vi "PDM Acq Cfg Popup.vi"(8 "error in (no error)":errorcluster, 11 "config file in":path caption="Configuration File") -> (0 "error out":errorcluster, 2 "output setting":T3={"PDM clock rate"=3072000.0, "decimation factor"=64, "bit clock direction"=enum."In", "logic level"=enum."3.3 V"} {"decimation factor" items=["24"=24, "32"=32, "48"=48, "64"=64, "96"=96, "128"=128]; "PDM clock rate" format="%#_6p"}, 3 "config file out":path caption="Configuration File")   [LabVIEW 2022 SP3, in "Config Dialog.lvlib"]
uses:
  Config Dialog.lvlib
  controls/PDM/PDM input settings.ctl
  <vilib>/PDM Acquisition Toolkit/shared/controls/decimation order.ctl
  controls/bit clock direction.ctl
  <vilib>/PDM Acquisition Toolkit/host/Classes/Session/Controls/Logic Levels.ctl
  controls/logic level.ctl
  <vilib>/Utility/miscctls.llb/LVPointTypeDef.ctl
  <vilib>/PDM Acquisition Toolkit/shared/PDM Shared.lvlib
  <vilib>/PDM Acquisition Toolkit/host/Classes/Session/DecoderSession.lvclass
  input configuration file/input cfg file.lvlib
  input configuration file/PDM/PDM input cfg file.lvlib
panel:
  out "bit clock rate":dbl=25600.0 caption="Bit Clock Rate" format="%#_6pS/s"
  in  "Logic Level":T1
  in  "Decimation":u16(ring) caption="master clock source" items=["x24"=24, "x32"=32, "x48"=48, "x64"=64, "x96"=96, "x128"=128]
  in  "Bit Clock Direction":T2 caption="master clock source"
  in  "sample rate":dbl=25600.0 caption="Sampling rate" format="%#_6pS/s"
  in  "Save":bool
  # "PDM Input Configuration"
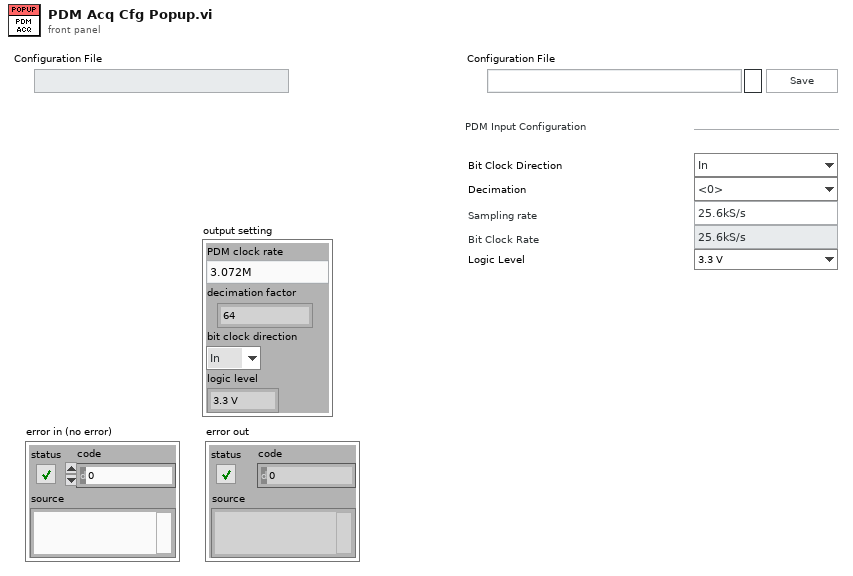
[diagram p1: front panel]
types:
  T1 = typedef "logic level.ctl" = enum32{"3.3 V", "1.8 V", "1.2 V"}
  T2 = typedef "bit clock direction.ctl" = enum32{"In", "Out"}
  T3 = typedef "PDM input settings.ctl" = cluster{"PDM clock rate":dbl, "decimation factor":T4, "bit clock direction":T2, "logic level":T5}
  T4 = typedef "PDM Shared.lvlib/decimation order.ctl" = u16
  T5 = typedef "PDM Acquisition Class Library.lvlib/DecoderSession.lvclass/Logic Levels.ctl" = enum16{"3.3 V", "1.8 V", "1.2 V"}
  T6 = typedef "LVPointTypeDef.ctl" = cluster{"Horizontal":i16, "Vertical":i16}
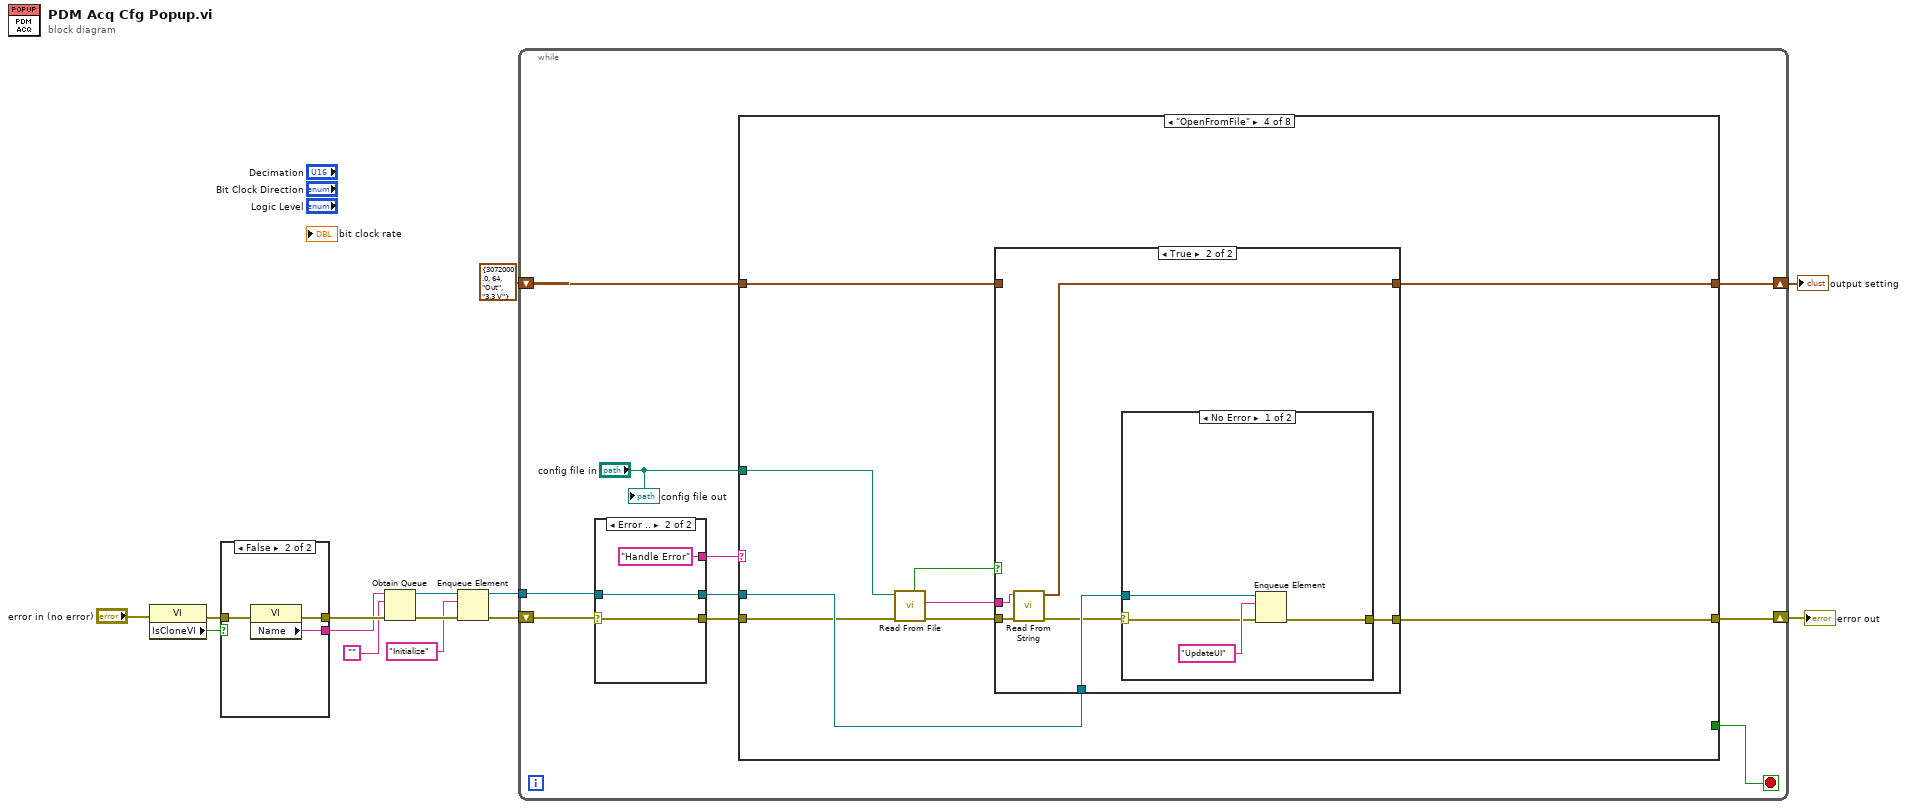
[diagram p0: block diagram]
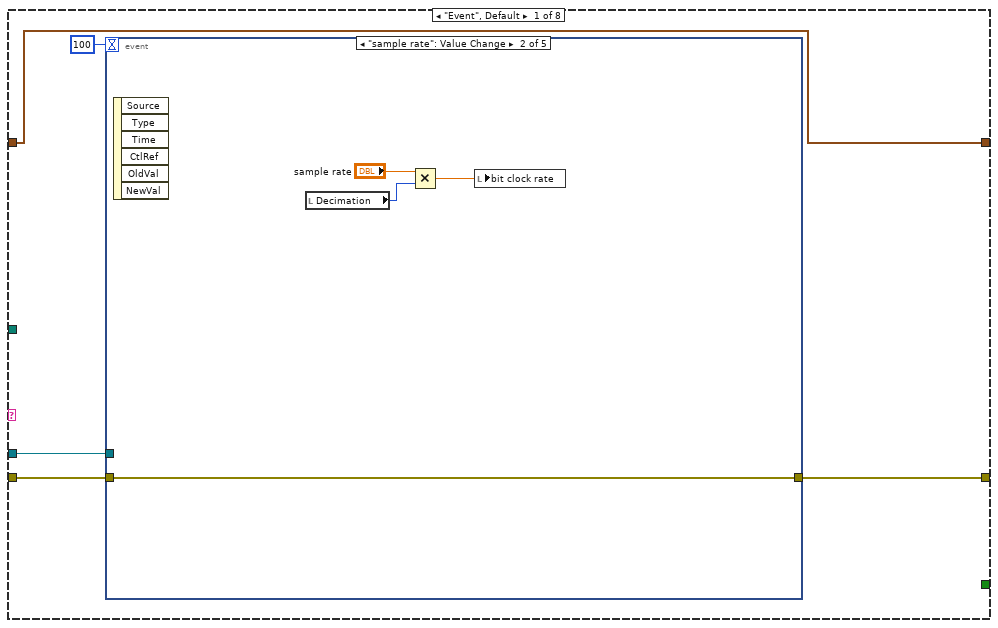
[diagram p2: hidden frame]
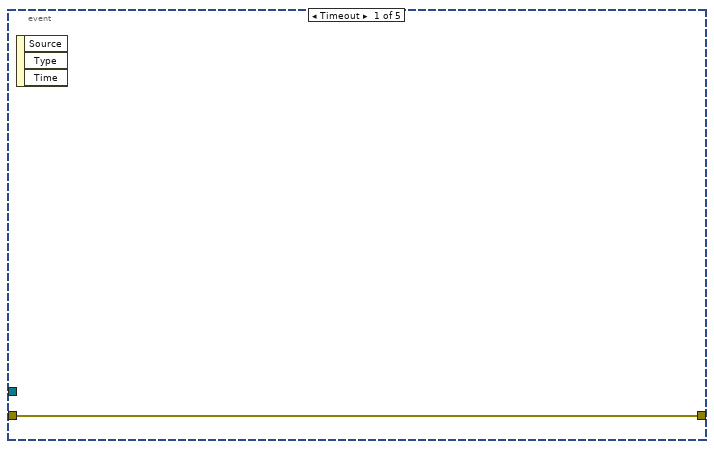
[diagram p3: hidden frame]
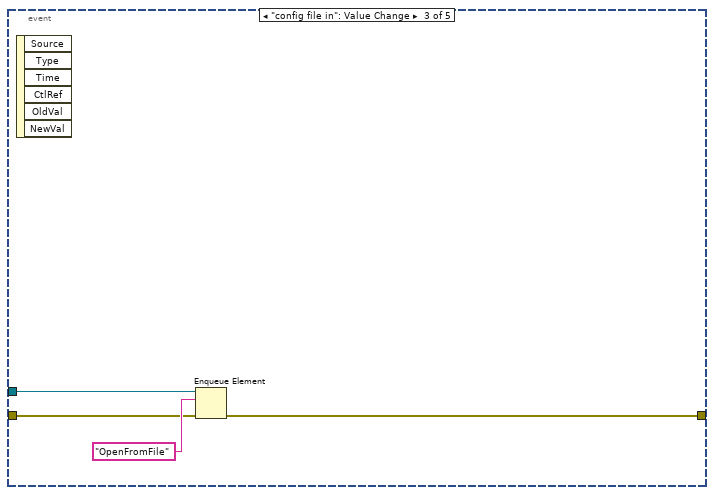
[diagram p4: hidden frame]
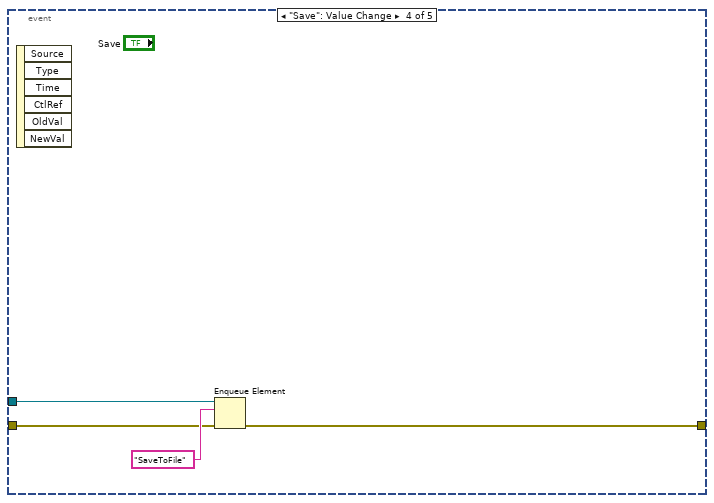
[diagram p5: hidden frame]
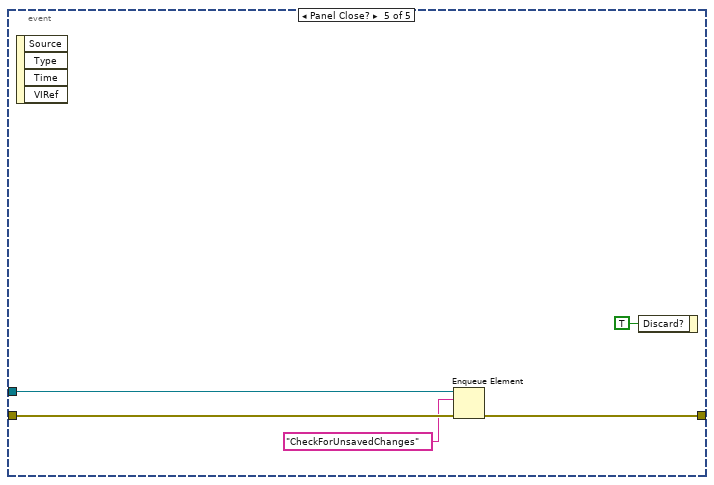
[diagram p6: hidden frame]
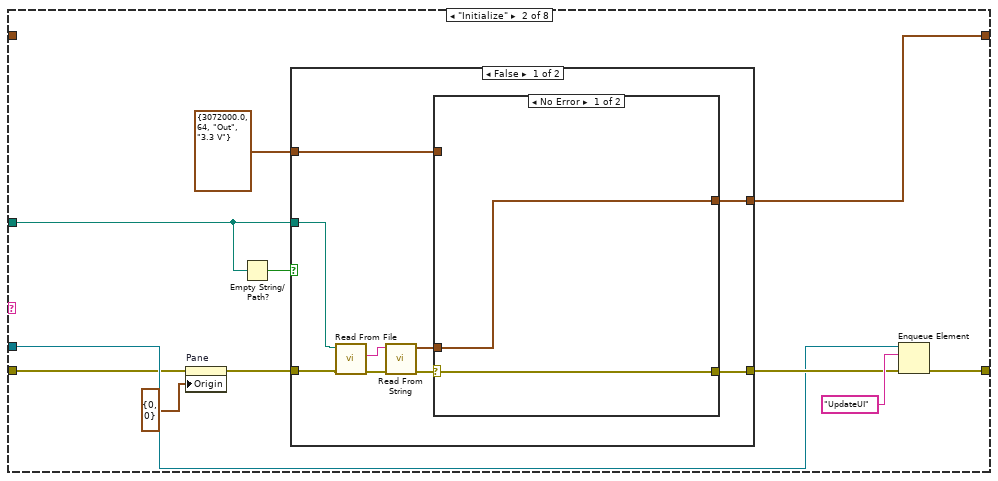
[diagram p7: hidden frame]
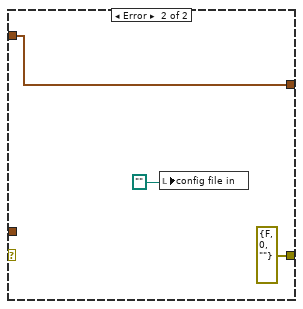
[diagram p8: hidden frame]
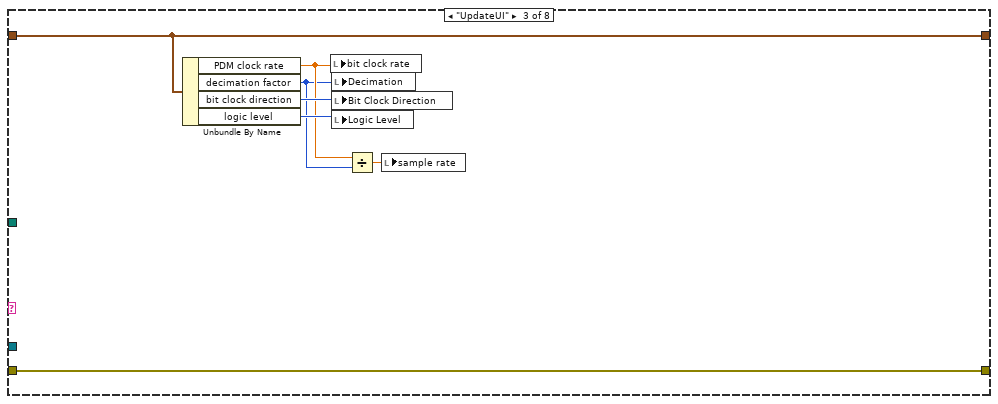
[diagram p10: hidden frame]
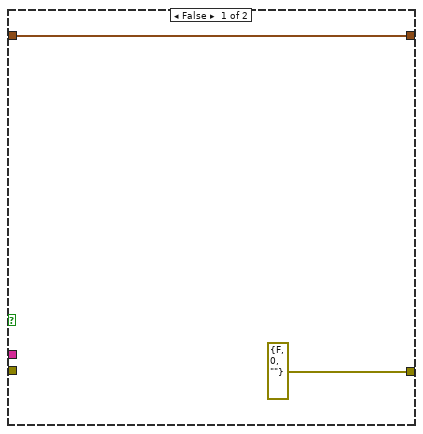
[diagram p11: hidden frame]
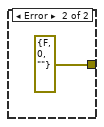
[diagram p12: hidden frame]
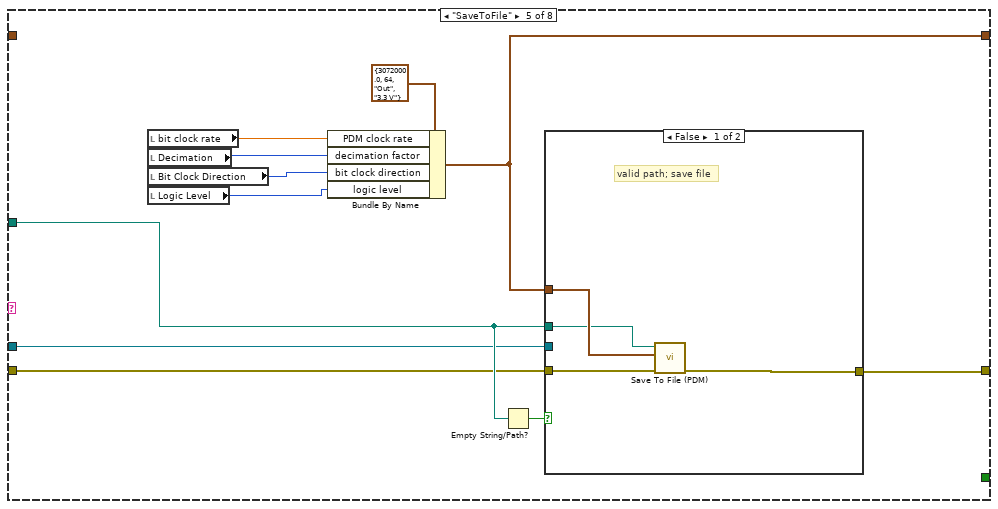
[diagram p13: hidden frame]
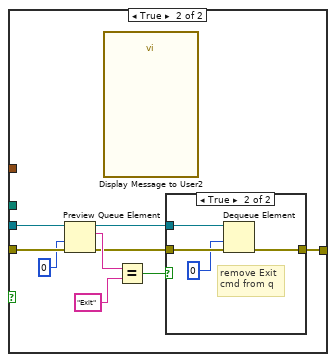
[diagram p14: hidden frame]
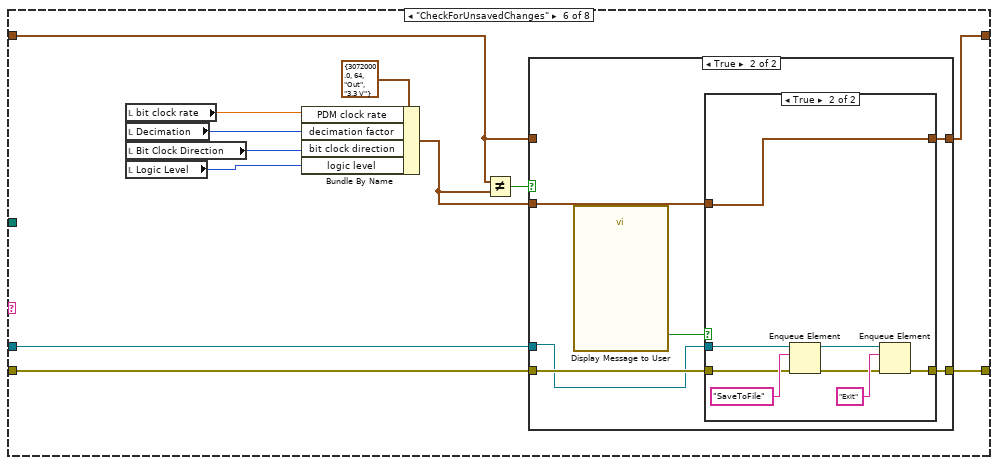
[diagram p16: hidden frame]
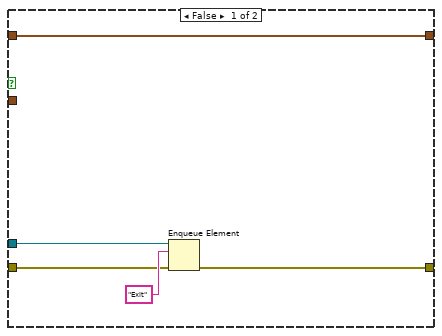
[diagram p17: hidden frame]
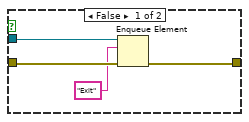
[diagram p18: hidden frame]
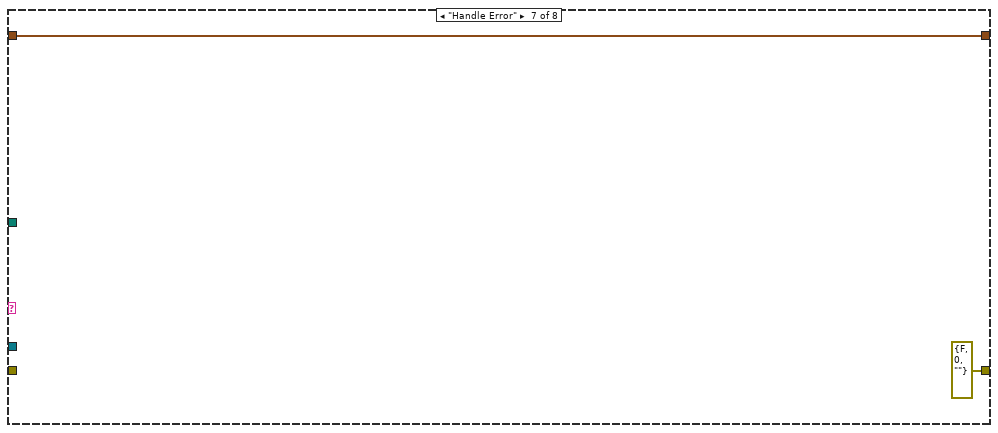
[diagram p19: hidden frame]
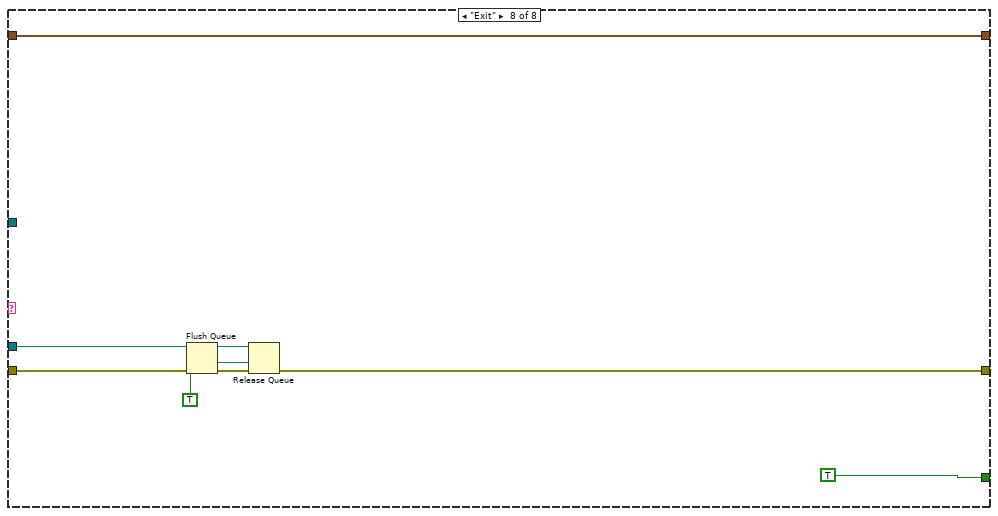
[diagram p20: hidden frame]
diagram:
  n1 = property class="VI"(error in="error in (no error)") -> (error out=w7:errorcluster, "IsCloneVI"=w8:bool)  [unwired: 1 in, 1 out]
  n2 = case shown="False" w8 {
    tunnel: [w17 w20] -> w14
    tunnel: [w16 w19] -> w13
    tunnel: w7 -> [w15 w18]
    frame True {
      n3 = property class="VI"(error in=w15) -> (error out=w17:errorcluster, "Clone Name"=w16:string)  [unwired: 1 in, 1 out]
    }
    frame False {
      n4 = property class="VI"(error in=w18) -> (error out=w20:errorcluster, "Name"=w19:string)  [unwired: 1 in, 1 out]
    }
  }
  n5 = Obtain Queue(name (unnamed)=w13, element data type="", error in (no error)=w14) -> (queue out=w11:refnum<queue>, error out=w12:errorcluster)  [unwired: 2 in, 1 out]
  n6 = Enqueue Element(queue=w11, element="Initialize", error in (no error)=w12) -> (queue out=w5:refnum<queue>, error out=w6:errorcluster)  [unwired: 1 in, 1 out]
  n7 = while {
    tunnel: w5 -> [w29]
    shift-right: [w25] -> w4
    shift-left: w6 -> [w30]
    shift-right: [w22] -> w1
    shift-left: T3 {"PDM clock rate"=3072000.0, "decimation factor"=64, "bit clock direction"=enum."Out", "logic level"=enum."3.3 V"} ("PDM input settings") -> [w23]
    stop <- w24 stop-if-true
    n8 = case shown="Error .." w30 {
      selector: w30 -> [w189 w192]
      tunnel: [w188 w192] -> w26
      tunnel: w29 -> [w187 w191]
      tunnel: [w186 w191] -> w27
      tunnel: [w185 "Handle Error"] -> w28
      frame No Error {
        n9 = Dequeue Element(queue=w187, timeout in ms (-1)=100, error in (no error)=w189) -> (queue out=w186:refnum<queue>, element=w185:string, error out=w188:errorcluster)  [unwired: 1 out]
      }
      frame Error {
      }
    }
    n10 = case shown="\"OpenFromFile\"" w28 {
      tunnel: w27 -> [w33 w58 _ w96 w115 w146 _ w179]
      tunnel: w26 -> [w34 w56 w87 w92 w117 w149 _ w180]
      tunnel: [w32 w59 w87 w95 w120 w148 errorcluster {"status"=FALSE, "code"=0, "source"=""} ("error out") w177] -> w25
      tunnel: [_ _ _ _ _ _ _ TRUE] -> w24
      tunnel: w23 -> [w31 _ w86 w94 _ w144 w175 w176]
      tunnel: [w31 w62 w86 w93 w119 w147 w175 w176] -> w22
      tunnel: "config file in" -> [_ w63 _ w91 w118 _ _ _]
      frame "Event", Default {
        n11 = event shown="[1] \"sample rate\": Value Change" {
          selector: _ -> [_ _ _ _ _]
          dyn-events: _ -> [_ _ _ _ _]
          timeout: 100 -> [_ _ _ _ _]
          tunnel: w34 -> [w36 w37 w43 w47 w52]
          tunnel: w33 -> [_ _ w42 w46 w51]
          tunnel: [w36 w37 w41 w45 w50] -> w32
          event Timeout {
            n12 = event-data() -> ()  [unwired: 1 in, 3 out]
          }
          event "sample rate": Value Change {
            n13 = event-data() -> ()  [unwired: 1 in, 6 out]
            n14 = local read "Decimation"() -> (w39:u16)
            n15 = Multiply(x="sample rate", y=w39) -> (x*y=w38:dbl)
            n16 = local write "bit clock rate"(w38) -> ()
          }
          event "config file in": Value Change {
            n17 = event-data() -> ()  [unwired: 1 in, 6 out]
            n18 = Enqueue Element(queue=w42, element="OpenFromFile", error in (no error)=w43) -> (error out=w41:errorcluster)  [unwired: 1 in, 2 out]
          }
          event "Save": Value Change {
            n19 = event-data() -> ()  [unwired: 1 in, 6 out]
            n20 = Enqueue Element(queue=w46, element="SaveToFile", error in (no error)=w47) -> (error out=w45:errorcluster)  [unwired: 1 in, 2 out]
          }
          event Panel Close? {
            n21 = event-data() -> ()  [unwired: 1 in, 4 out]
            n22 = Enqueue Element(queue=w51, element="CheckForUnsavedChanges", error in (no error)=w52) -> (error out=w50:errorcluster)  [unwired: 1 in, 2 out]
            n23 = event-data("Discard?"=TRUE) -> ()  [unwired: 1 in, 1 out]
          }
        }
      }
      frame "Initialize" {
        n24 = property on="Pane" class="Pane"(error in=w56, "Origin"=T6 {"Horizontal"=0, "Vertical"=0}) -> (error out=w55:errorcluster)  [unwired: 1 in, 1 out]
        n25 = Empty String/Path?(string/path=w63) -> (empty?=w64:bool)
        n26 = case shown="False" w64 {
          tunnel: w55 -> [w70 w80]
          tunnel: w63 -> [w69 _]
          tunnel: [w71 w79] -> w62
          tunnel: [w73 w80] -> w60
          tunnel: T3 {"PDM clock rate"=3072000.0, "decimation factor"=64, "bit clock direction"=enum."Out", "logic level"=enum."3.3 V"} ("PDM input settings") -> [w72 w79]
          frame False {
            n27 = call "Read From File.vi"("error in (no error)"=w70, "file path"=w69) -> ("error out"=w68:errorcluster, "input cfg JSON"=w65:string)  [unwired: 6 in, 2 out]
            n28 = call "Read From String.vi"("error in (no error)"=w68, "JSON string"=w65) -> ("error out"=w67:errorcluster, "input settings"=w66:T3)  [unwired: 8 in]
            n29 = case shown="No Error" w67 {
              selector: w67 -> [w74 _]
              tunnel: w66 -> [w75 _]
              tunnel: [w75 w76] -> w71
              tunnel: [w74 errorcluster {"status"=FALSE, "code"=0, "source"=""} ("error IO")] -> w73
              tunnel: w72 -> [_ w76]
              frame No Error {
              }
              frame Error {
                n30 = local write "config file in"(path "") -> ()
              }
            }
          }
          frame True {
          }
        }
        n31 = Enqueue Element(queue=w58, element="UpdateUI", error in (no error)=w60) -> (error out=w59:errorcluster)  [unwired: 1 in, 2 out]
      }
      frame "UpdateUI" {
        n32 = Unbundle By Name(w86) -> ("PDM clock rate"=w83:dbl, "decimation factor"=w82:T4, "bit clock direction"=w85:T2, "logic level"=w84:T5)
        n33 = local write "bit clock rate"(w83) -> ()
        n34 = local write "Decimation"(w82) -> ()
        n35 = local write "Bit Clock Direction"(w85) -> ()
        n36 = local write "Logic Level"(w84) -> ()
        n37 = Divide(x=w83, y=w82) -> (x/y=w81:dbl)
        n38 = local write "sample rate"(w81) -> ()
      }
      frame "OpenFromFile" {
        n39 = call "Read From File.vi"("error in (no error)"=w92, "file path"=w91) -> ("error out"=w89:errorcluster, "input cfg JSON"=w88:string, "file exists?"=w90:bool)  [unwired: 6 in, 1 out]
        n40 = case shown="True" w90 {
          tunnel: w96 -> [_ w104]
          tunnel: [errorcluster {"status"=FALSE, "code"=0, "source"=""} ("error out") w103] -> w95
          tunnel: w94 -> [w98 _]
          tunnel: [w98 w100] -> w93
          tunnel: w89 -> [_ w102]
          tunnel: w88 -> [_ w99]
          frame False {
          }
          frame True {
            n41 = call "Read From String.vi"("error in (no error)"=w102, "JSON string"=w99) -> ("error out"=w101:errorcluster, "input settings"=w100:T3)  [unwired: 8 in]
            n42 = case shown="No Error" w101 {
              selector: w101 -> [w105 _]
              tunnel: w104 -> [w107 _]
              tunnel: [w106 errorcluster {"status"=FALSE, "code"=0, "source"=""} ("error out")] -> w103
              frame No Error {
                n43 = Enqueue Element(queue=w107, element="UpdateUI", error in (no error)=w105) -> (error out=w106:errorcluster)  [unwired: 1 in, 2 out]
              }
              frame Error {
              }
            }
          }
        }
      }
      frame "SaveToFile" {
        n44 = local read "bit clock rate"() -> (w114:dbl)
        n45 = local read "Decimation"() -> (w113:u16)
        n46 = local read "Bit Clock Direction"() -> (w112:T2)
        n47 = local read "Logic Level"() -> (w110:T1)
        n48 = Bundle By Name(cluster=T3 {"PDM clock rate"=3072000.0, "decimation factor"=64, "bit clock direction"=enum."Out", "logic level"=enum."3.3 V"} ("PDM input settings"), "PDM clock rate"=w114, "decimation factor"=w113, "bit clock direction"=w112, "logic level"=w110) -> (w119:T3)
        n49 = Empty String/Path?(string/path=w118) -> (empty?=w116:bool)
        n50 = case shown="False" w116 {
          tunnel: [w123 w126] -> w120
          tunnel: w119 -> [w122 _]
          tunnel: w118 -> [w121 _]
          tunnel: w117 -> [w124 w133]
          tunnel: w115 -> [_ w132]
          frame False {
            # "valid path; save file"
            n51 = call "Save To File (PDM).vi"("error in (no error)"=w124, "PDM input settings"=w122, "file path"=w121) -> ("error out"=w123:errorcluster)  [unwired: 8 in]
          }
          frame True {
            n52 = Preview Queue Element(queue=w132, timeout in ms (-1)=0, error in (no error)=w133) -> (queue out=w129:refnum<queue>, element=w131:string, error out=w127:errorcluster)  [unwired: 1 out]
            n53 = call "Display Message to User2"() -> ()  [unwired: 10 in, 2 out]
            n54 = Equal?(x=w131, y="Exit") -> (x = y?=w128:bool)
            n55 = case shown="True" w128 {
              tunnel: w129 -> [_ w138]
              tunnel: w127 -> [w134 w137]
              tunnel: [w134 w136] -> w126
              frame False {
              }
              frame True {
                # "remove Exit\ncmd from q"
                n56 = Dequeue Element(queue=w138, timeout in ms (-1)=0, error in (no error)=w137) -> (error out=w136:errorcluster)  [unwired: 3 out]
              }
            }
          }
        }
      }
      frame "CheckForUnsavedChanges" {
        n57 = local read "bit clock rate"() -> (w141:dbl)
        n58 = local read "Decimation"() -> (w142:u16)
        n59 = local read "Bit Clock Direction"() -> (w143:T2)
        n60 = local read "Logic Level"() -> (w139:T1)
        n61 = Bundle By Name(cluster=T3 {"PDM clock rate"=3072000.0, "decimation factor"=64, "bit clock direction"=enum."Out", "logic level"=enum."3.3 V"} ("PDM input settings"), "PDM clock rate"=w141, "decimation factor"=w142, "bit clock direction"=w143, "logic level"=w139) -> (w145:T3)
        n62 = Not Equal?(x=w144, y=w145) -> (x != y?=w150:bool)
        n63 = case shown="True" w150 {
          tunnel: w149 -> [w153 w161]
          tunnel: [w151 w157] -> w148
          tunnel: w145 -> [_ w159]
          tunnel: w144 -> [w155 _]
          tunnel: [w155 w158] -> w147
          tunnel: w146 -> [w152 w156]
          frame False {
            n64 = Enqueue Element(queue=w152, element="Exit", error in (no error)=w153) -> (error out=w151:errorcluster)  [unwired: 1 in, 2 out]
          }
          frame True {
            n65 = call "Display Message to User"() -> ("Yes"=w160:bool)  [unwired: 10 in, 1 out]
            n66 = case shown="True" w160 {
              tunnel: w161 -> [w165 w172]
              tunnel: w159 -> [_ w171]
              tunnel: [_ w171] -> w158
              tunnel: [w163 w167] -> w157
              tunnel: w156 -> [w164 w166]
              frame False {
                n67 = Enqueue Element(queue=w164, element="Exit", error in (no error)=w165) -> (error out=w163:errorcluster)  [unwired: 1 in, 2 out]
              }
              frame True {
                n68 = Enqueue Element(queue=w166, element="SaveToFile", error in (no error)=w172) -> (queue out=w168:refnum<queue>, error out=w169:errorcluster)  [unwired: 1 in, 1 out]
                n69 = Enqueue Element(queue=w168, element="Exit", error in (no error)=w169) -> (error out=w167:errorcluster)  [unwired: 1 in, 2 out]
              }
            }
          }
        }
      }
      frame "Handle Error" {
      }
      frame "Exit" {
        n70 = Flush Queue(queue=w179, error in (no error)=w180) -> (queue out=w183:refnum<queue>, error out=w182:errorcluster)  [unwired: 1 out]
        n71 = Release Queue(queue=w183, force destroy? (F)=TRUE, error in (no error)=w182) -> (error out=w177:errorcluster)  [unwired: 2 out]
      }
    }
    "config file out" <- "config file in"
  }
  "error out" <- w4
  "output setting" <- w1
